vi "GetEcalInfo.vi"(8 "error in (no error)":errorcluster, 11 "NetA_AgNA in":refnum<class "NetA_AgNA.lvclass">) -> (0 "error out":errorcluster, 2 "ECal Info":string, 3 "NetA_AgNA out":refnum<class "NetA_AgNA.lvclass">)   [LabVIEW 2014, in "NetA_AgNA.lvclass"]
doc: "Returns ecal information. Does not require knowledge of the connectors."
uses:
  NetA_AgNA.lvclass
  NetA_AgNA.lvclass/NetA_AgNA.ctl
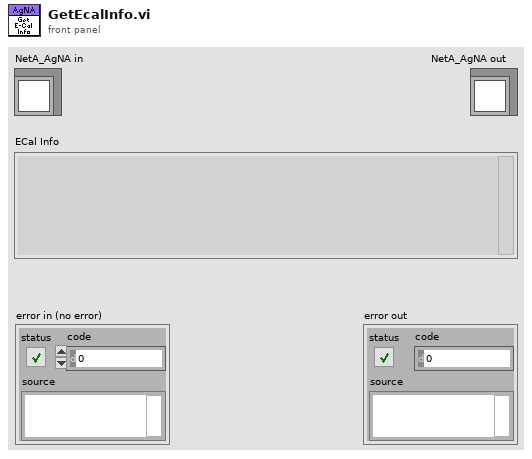
[diagram p1: front panel]
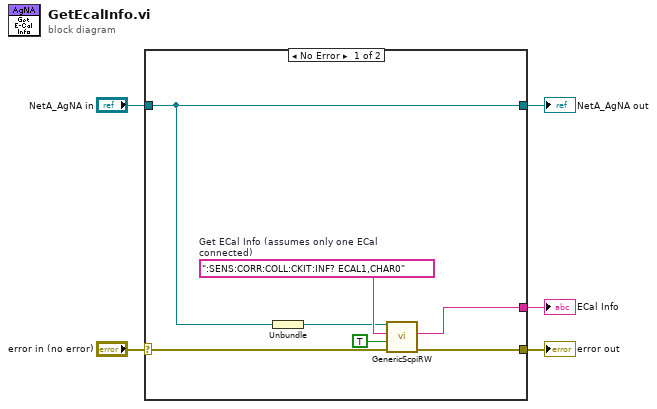
[diagram p0: block diagram]
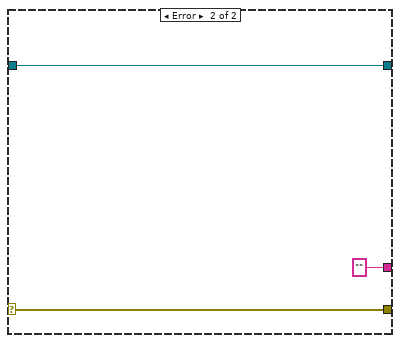
[diagram p2: hidden frame]
diagram:
  n1 = case shown="No Error" "error in (no error)" {
    selector: "error in (no error)" -> [w11 w14]
    tunnel: [w12 w14] -> w5
    tunnel: [w8 "" ("SCPI Response")] -> w3
    tunnel: "NetA_AgNA in" -> [w7 w15]
    tunnel: [w7 w15] -> w1
    frame No Error {
      w10 = ":SENS:CORR:COLL:CKIT:INF? ECAL1,CHAR0"  # Get ECal Info (assumes only one ECal connected)
      n2 = Unbundle(w7) -> (w6:refnum<k15>)
      n3 = call "GenericScpiRW.vi"("error in (no error)"=w11, "Query?"=TRUE, "SCPI Command"=w10, "resource name"=w6) -> ("error out"=w12:errorcluster, "SCPI Response"=w8:string)  [unwired: 6 in]
    }
    frame Error {
    }
  }
  "ECal Info" <- w3
  "error out" <- w5
  "NetA_AgNA out" <- w1
